vi "Symbol Upload Info.vi"(8 "Error In":errorcluster, 11 "AMS Connection In":T1) -> (0 "Error Out":errorcluster, 2 "Symsize":u32, 3 "Symbols":u32)   [LabVIEW 2017, in "TwinCAT ADS.lvlib" / "PLC.lvlib"]
uses:
  PLC.lvlib
  Low Level/TypeDefs/AMS Connection.ctl
  Low Level/TypeDefs/AMS.ctl
  TwinCAT ADS.lvlib
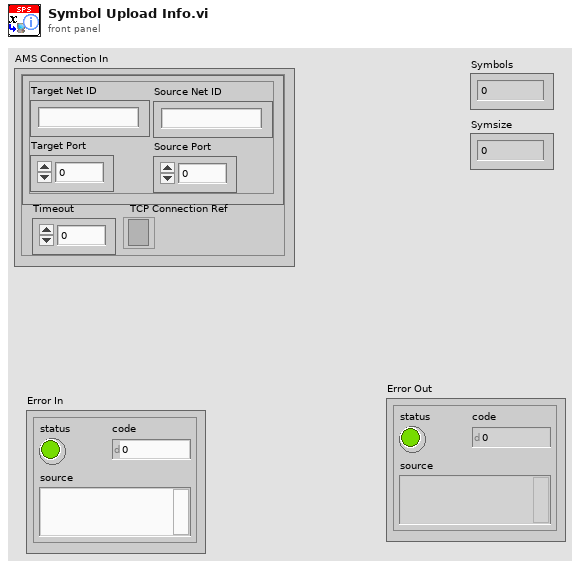
[diagram p1: front panel]
types:
  T1 = typedef "TwinCAT ADS.lvlib/AMS Connection.ctl" = cluster{"AMS":T2, "Timeout":i32, "TCP Connection Ref":refnum<k5>}
  T2 = typedef "TwinCAT ADS.lvlib/AMS.ctl" = cluster{"Target Net ID":string, "Target Port":u16, "Source Net ID":string, "Source Port":u16}
  T3 = typedef "TwinCAT ADS.lvlib/ADS Error.ctl" = i32
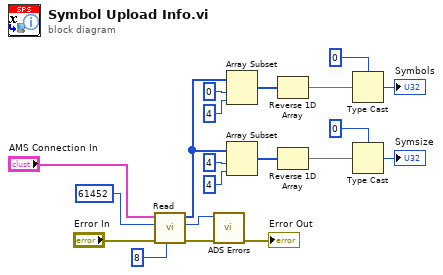
[diagram p0: block diagram]
diagram:
  n1 = call "Read.vi"("Read Length"=u32 8, "Error In"="Error In", "Index Group"=u32 61452, "AMS Connection In"="AMS Connection In") -> ("Error Out"=w2:errorcluster, "ADS Error"=w3:T3, "Data"=w4:u8[])  [unwired: 5 in]
  n2 = call "ADS Errors.vi"("error in (no error)"=w2, "ADS Error"=w3) -> ("error out"=→"Error Out":errorcluster)  [unwired: 9 in]
  n3 = Array Subset(array=w4, index=0, length=4) -> (w16:u8[])
  n4 = Array Subset(array=w4, index=4, length=4) -> (w12:u8[])
  n5 = Reverse 1D Array(array=w16) -> (reversed array=w8:u8[])
  n6 = Reverse 1D Array(array=w12) -> (reversed array=w7:u8[])
  n7 = Type Cast(type=u32 0, x=w8) -> (*(type *) &x=→"Symbols":u32)
  n8 = Type Cast(type=u32 0, x=w7) -> (*(type *) &x=→"Symsize":u32)
